vi "defer panel updates.vi"(8 "error in (no error)":errorcluster, 10 "defer? (F)":bool, 11 "vi ref":refnum<vi>) -> (0 "error out":errorcluster)   [LabVIEW 2024, in "controls manager.lvlib"]
uses:
  controls manager.lvlib
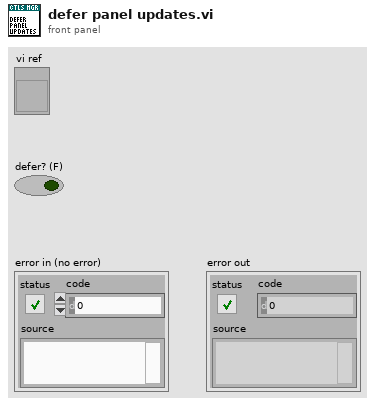
[diagram p1: front panel]
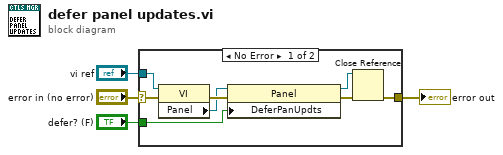
[diagram p0: block diagram]
diagram:
  n1 = case shown="No Error" "error in (no error)" {
    selector: "error in (no error)" -> [w6 w13]
    tunnel: "defer? (F)" -> [w11 _]
    tunnel: "vi ref" -> [w10 _]
    tunnel: [w7 w13] -> w1
    frame No Error {
      n2 = property class="VI"(reference=w10, error in=w6) -> (error out=w8:errorcluster, "Panel"=w5:refnum<vi>)  [unwired: 1 out]
      n3 = property class="Panel"(reference=w5, error in=w8, "DeferPanUpdts"=w11) -> (reference out=w9:refnum<vi>, error out=w12:errorcluster)
      n4 = Close Reference(reference=w9, error in (no error)=w12) -> (error out=w7:errorcluster)
    }
    frame Error {
    }
  }
  "error out" <- w1
